vi "X sensor convert V to meter.vi"(10 "Sensor X Voltage":dbl) -> (2 "X coordinate":dbl format="%#_6p")   [LabVIEW 2013]
doc: "This VI convert the X piezo from Voltage to actual displacement um."
uses:
  <vilib>/Levylab/General AFM Lithography/subvi/Drivers/Cypher XY LVDT Parameters.vi
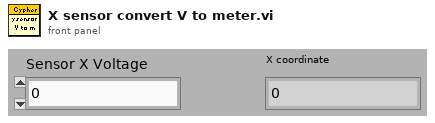
[diagram p1: front panel]
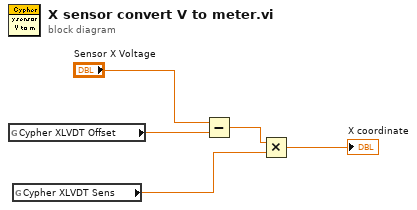
[diagram p0: block diagram]
diagram:
  n1 = global read "Cypher XY LVDT Parameters.vi" "Cypher XLVDT Offset"() -> (w4:dbl)
  n2 = global read "Cypher XY LVDT Parameters.vi" "Cypher XLVDT Sens"() -> (w3:dbl)
  n3 = Subtract(x="Sensor X Voltage", y=w4) -> (x-y=w2:dbl)
  n4 = Multiply(x=w2, y=w3) -> (x*y=→"X coordinate":dbl)
